vi "FT_Get_Device_Description_By_Index.vi"(8 "error in (no error)":errorcluster, 11 "Device Index":u32) -> (0 "error out":errorcluster, 1 "FT_Status":u32(ring) items=["FT_OK", "FT_INVALID_HANDLE", "FT_DEVICE_NOT_FOUND", "FT_DEVICE_NOT_OPENED", "FT_IO_ERROR", "FT_INSUFFICIENT_RESOURCES", "FT_INVALID_PARAMETER", "FT_INVALID_BAUD_RATE", "FT_DEVICE_NOT_OPENED_FOR_ERASE", "FT_DEVICE_NOT_OPENED_FOR_WRITE", "FT_FAILED_TO_WRITE_DEVICE", "FT_EEPROM_READ_FAILED", "FT_EEPROM_WRITE_FAILED", "FT_EEPROM_ERASE_FAILED", "FT_EEPROM_NOT_PRESENT", "FT_EEPROM_NOT_PROGRAMMED", "FT_INVALID_ARGS", "FT_NOT_SUPPORTED", "FT_OTHER_ERROR"], 3 "Device Description":string)   [LabVIEW 2018]
uses:
  FTD2XX.dll
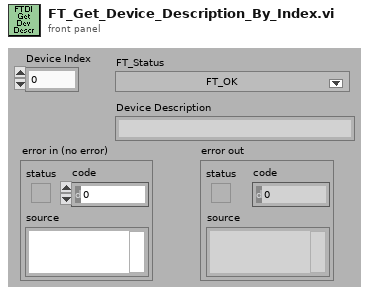
[diagram p1: front panel]
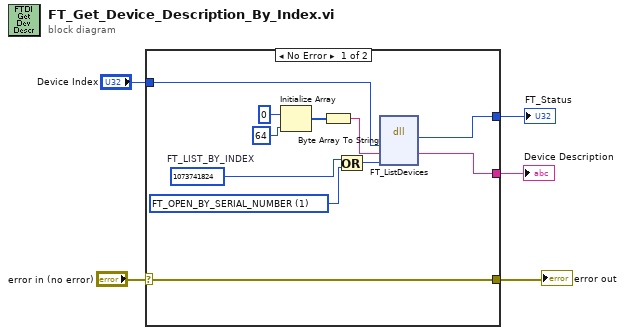
[diagram p0: block diagram]
diagram:
  n1 = case shown="No Error" "error in (no error)" {
    selector: "error in (no error)" -> [w6 w17]
    tunnel: [w16 _] -> w5
    tunnel: [w15 _] -> w4
    tunnel: "Device Index" -> [w14 _]
    tunnel: [w6 w17] -> w1
    frame No Error {
      w13 = u32 1 items=["FT_OPEN_BY_SERIAL_NUMBER"=1, "FT_OPEN_BY_DESCRIPTION"=2, "FT_OPEN_BY_LOCATION"=4] ("Flags")
      w12 = u32 1073741824  # FT_LIST_BY_INDEX
      n2 = Initialize Array(u8 0, 64 ("dimension size")) -> (w9:u8[])
      n3 = Byte Array To String(unsigned byte array=w9) -> (string=w8:string)
      n4 = Or(x=w12, y=w13) -> (x .or. y?=w11:u32)
      n5 = dll-call lib="FTD2XX.dll" fn="FT_ListDevices"("DeviceIndex"=w14, "DeviceDescription"=w8, "Flags"=w11) -> ("FT_Status"=w16:u32, "DeviceDescription"=w15:string)  [unwired: 5 in, 2 out]
    }
    frame Error {
    }
  }
  "FT_Status" <- w5
  "Device Description" <- w4
  "error out" <- w1
